vi "Read Observation Title.vi"(8 "error in (no error)":errorcluster, 11 "Save Image in":refnum<class "Save Image.lvclass">) -> (0 "error out":errorcluster, 2 "OBS_TITLE.Value":string, 3 "Save Image out":refnum<class "Save Image.lvclass">)   [LabVIEW 2018, in "Save Image.lvclass"]
uses:
  Save Image.lvclass
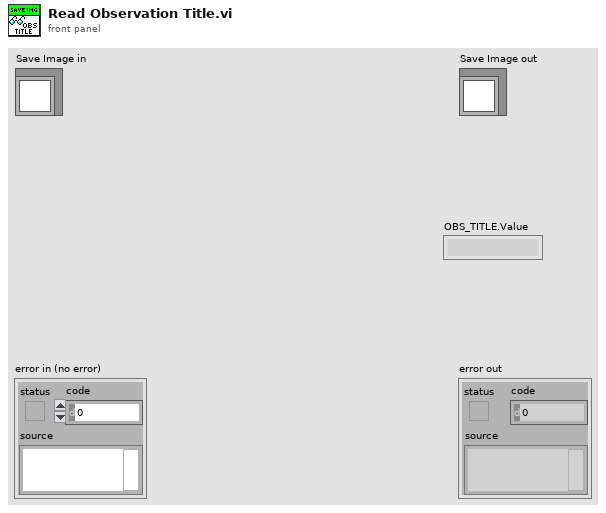
[diagram p1: front panel]
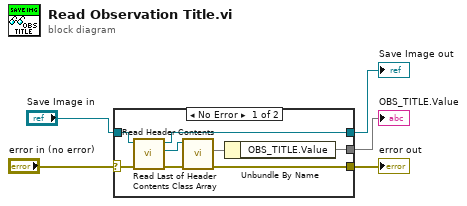
[diagram p0: block diagram]
diagram:
  n1 = case shown="No Error" "error in (no error)" {
    selector: "error in (no error)" -> [w6 w15]
    tunnel: [w8 w15] -> w4
    tunnel: [w9 w14] -> w2
    tunnel: "Save Image in" -> [w11 w14]
    tunnel: [w13 _] -> w1
    frame No Error {
      n2 = call "Read Last of Header Contents Class Array.vi"("error in (no error)"=w6, "Save Image in"=w11) -> ("error out"=w7:errorcluster, "Simulated_Header.lvclass"=w10:refnum<class "Simulated_Header.lvclass">, "Save Image out"=w9:refnum<class "Save Image.lvclass">)  [unwired: 7 in]
      n3 = call "Read Header Contents.vi"("error in (no error)"=w7, "Header in"=w10) -> ("error out"=w8:errorcluster, 2:w12)  [unwired: 7 in, 1 out]
      n4 = Unbundle By Name(w12) -> ("OBS_TITLE.Value"=w13)
    }
    frame Error {
    }
  }
  "error out" <- w4
  "Save Image out" <- w2
  "OBS_TITLE.Value" <- w1
